vi "Read Data.vi"(8 "error in (no error)":errorcluster, 10 "Send Command (Empty)":string, 11 "VISA resource name":refnum<visa-resource-name>) -> (0 "error out":errorcluster, 1 "Data Length":i32, 2 "Read Data":string, 3 "VISA resource name out":refnum<visa-resource-name>)   [LabVIEW 2019, in "Yokogawa WT300 Series.lvlib"]
doc: "Writes the string data and receives a maximum of bytes to read bytes from the specified interface connection, returning the results in Read Data."
uses:
  Yokogawa WT300 Series.lvlib
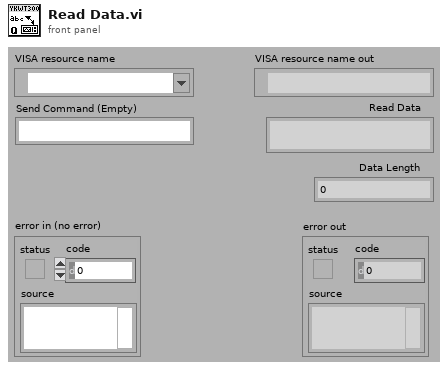
[diagram p1: front panel]
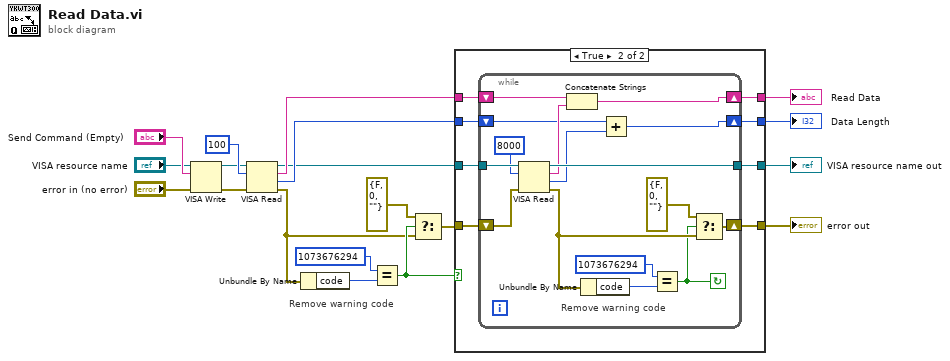
[diagram p0: block diagram]
diagram:
  # "Remove warning code"
  n1 = VISA Write(VISA resource name="VISA resource name", write buffer="Send Command (Empty)", error in (no error)="error in (no error)") -> (VISA resource name out=w8:refnum<visa-resource-name>, error out=w9:errorcluster)  [unwired: 1 out]
  n2 = VISA Read(VISA resource name=w8, byte count=u32 100, error in (no error)=w9) -> (VISA resource name out=w10:refnum<visa-resource-name>, read buffer=w19:string, return count=w18:u32, error out=w15:errorcluster)
  n3 = Unbundle By Name(w15) -> ("code"=w11:i32)
  n4 = Equal?(x=1073676294, y=w11) -> (x = y?=w16:bool)
  n5 = Select(t=errorcluster {"status"=FALSE, "code"=0, "source"=""}, s=w16, f=w15) -> (s? t:f=w14:errorcluster)
  n6 = case shown="True" w16 {
    tunnel: w10 -> [w23 w31]
    tunnel: w14 -> [w22 w28]
    tunnel: [w23 w30] -> w2
    tunnel: [w22 w29] -> w1
    tunnel: w18 -> [w20 w27]
    tunnel: [w21 w26] -> w7
    tunnel: w19 -> [w21 w25]
    tunnel: [w20 w24] -> w6
    frame False {
    }
    frame True {
      n7 = while {
        shift-left: w28 -> [w42]
        shift-right: [w33] -> w29
        shift-left: w25 -> [w44]
        shift-right: [w45] -> w26
        shift-left: w27 -> [w41]
        shift-right: [w39] -> w24
        tunnel: [w46] -> w30
        tunnel: w31 -> [w47]
        stop <- w32 continue-if-true
        # "Remove warning code"
        n8 = VISA Read(VISA resource name=w47, byte count=u32 8000, error in (no error)=w42) -> (VISA resource name out=w46:refnum<visa-resource-name>, read buffer=w43:string, return count=w40:u32, error out=w34:errorcluster)
        n9 = Concatenate Strings(w44, w43) -> (w45:string)
        n10 = Unbundle By Name(w34) -> ("code"=w37:i32)
        n11 = Add(x=w41, y=w40) -> (x+y=w39:u32)
        n12 = Equal?(x=1073676294, y=w37) -> (x = y?=w32:bool)
        n13 = Select(t=errorcluster {"status"=FALSE, "code"=0, "source"=""}, s=w32, f=w34) -> (s? t:f=w33:errorcluster)
      }
    }
  }
  "error out" <- w1
  "VISA resource name out" <- w2
  "Data Length" <- w6
  "Read Data" <- w7
